vi "Analog Replay 1.0 Voltage Scaling.vi"(5 "Device Inputs":dbl[](array[numeric]), 6 "reset in":bool, 7 "Last Device Inputs":dbl[](array[numeric]), 8 "SE_VScaleSlope":fxp<+,18,6>, 9 "SE_VScaleIntercept":fxp<+/-,18,3>, 10 "input in":T1, 11 "FIFO indexes":T2) -> (1 "reset out":bool, 2 "input out":T1, 3 "write":bool)   [LabVIEW 2017, in "Engine Simulation Toolkit Engine.lvlib"]
uses:
  Engine Simulation Toolkit Engine.lvlib
  Shared/1.0 Analog Replay FIFO Idxs.ctl
  Shared/Engine Simulation Toolkit Shared.lvlib
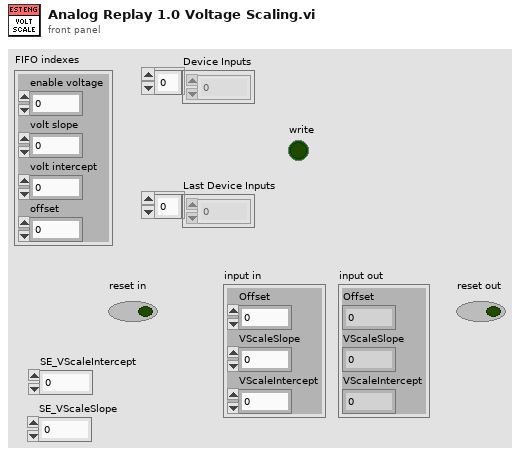
[diagram p1: front panel]
types:
  T1 = cluster{"Offset":i16, "VScaleSlope":fxp<+,18,6>, "VScaleIntercept":fxp<+/-,18,3>}
  T2 = typedef "Engine Simulation Toolkit Shared.lvlib/1.0 Analog Replay FIFO Idxs.ctl" = cluster{"enable voltage":i32, "volt slope":i32, "volt intercept":i32, "offset":i32}
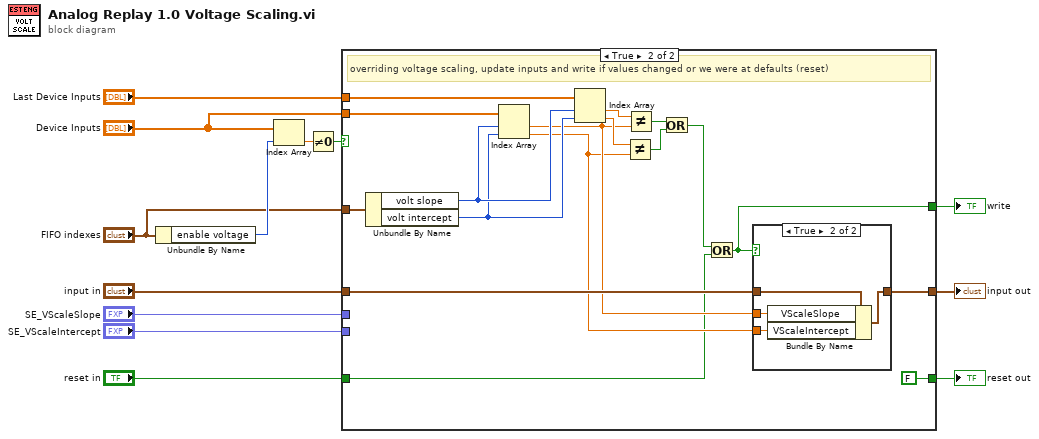
[diagram p0: block diagram]
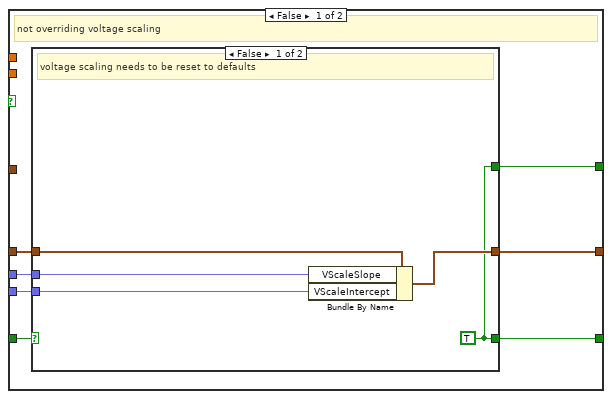
[diagram p2: hidden frame]
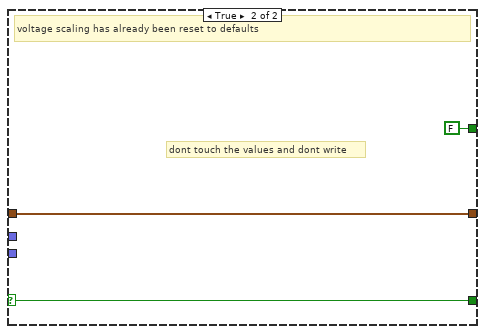
[diagram p3: hidden frame]
diagram:
  n1 = Unbundle By Name("FIFO indexes") -> ("enable voltage"=w13:i32)
  n2 = Index Array(array="Device Inputs", index=w13) -> (element=w12:dbl)
  n3 = Not Equal To 0?(x=w12) -> (x != 0?=w11:bool)
  n4 = case shown="True" w11 {
    tunnel: "input in" -> [w19 w34]
    tunnel: [w18 w33] -> w9
    tunnel: [w17 FALSE] -> w8
    tunnel: "SE_VScaleSlope" -> [w16 _]
    tunnel: "SE_VScaleIntercept" -> [w15 _]
    tunnel: [w14 w29] -> w5
    tunnel: "FIFO indexes" -> [_ w45]
    tunnel: "Last Device Inputs" -> [_ w44]
    tunnel: "Device Inputs" -> [_ w43]
    tunnel: "reset in" -> [w20 w30]
    frame False {
      # "not overriding voltage scaling"
      n5 = case shown="False" w20 {
        selector: w20 -> [_ w27]
        tunnel: w19 -> [w25 w28]
        tunnel: [w24 w28] -> w18
        tunnel: [w21 w27] -> w17
        tunnel: w16 -> [w23 _]
        tunnel: w15 -> [w22 _]
        tunnel: [w21 FALSE] -> w14
        frame False {
          w21 = TRUE
          # "voltage scaling needs to be reset to defaults"
          n6 = Bundle By Name(cluster=w25, "VScaleSlope"=w23, "VScaleIntercept"=w22) -> (w24:T1)
        }
        frame True {
          # "dont touch the values and dont write"
          # "voltage scaling has already been reset to defaults"
        }
      }
    }
    frame True {
      # "overriding voltage scaling, update inputs and write if values changed or we were at defaults (reset)"
      n7 = Unbundle By Name(w45) -> ("volt slope"=w42:i32, "volt intercept"=w41:i32)
      n8 = Index Array(array=w43, index #1=w42, index #2=w41) -> (element #1=w32:dbl, element #2=w31:dbl)
      n9 = Index Array(array=w44, index #1=w42, index #2=w41) -> (element #1=w40:dbl, element #2=w39:dbl)
      n10 = Not Equal?(x=w39, y=w31) -> (x != y?=w37:bool)
      n11 = Not Equal?(x=w40, y=w32) -> (x != y?=w38:bool)
      n12 = Or(x=w38, y=w37) -> (x .or. y?=w35:bool)
      n13 = Or(x=w35, y=w30) -> (x .or. y?=w29:bool)
      n14 = case shown="True" w29 {
        tunnel: w34 -> [w46 w50]
        tunnel: [w46 w49] -> w33
        tunnel: w32 -> [_ w48]
        tunnel: w31 -> [_ w47]
        frame False {
        }
        frame True {
          n15 = Bundle By Name(cluster=w50, "VScaleSlope"=w48, "VScaleIntercept"=w47) -> (w49:T1)
        }
      }
    }
  }
  "input out" <- w9
  "write" <- w5
  "reset out" <- w8
